vi "LogState.vi"(8 "error in (no error)":errorcluster, 10 "State In":string, 11 "String in":refnum<vi>) -> (0 "error out":errorcluster, 2 "State Out":string)   [LabVIEW 2017]
panel:
  out "Log line":string
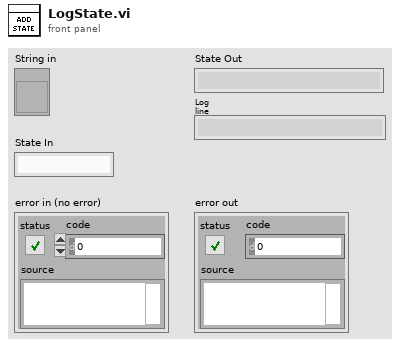
[diagram p1: front panel]
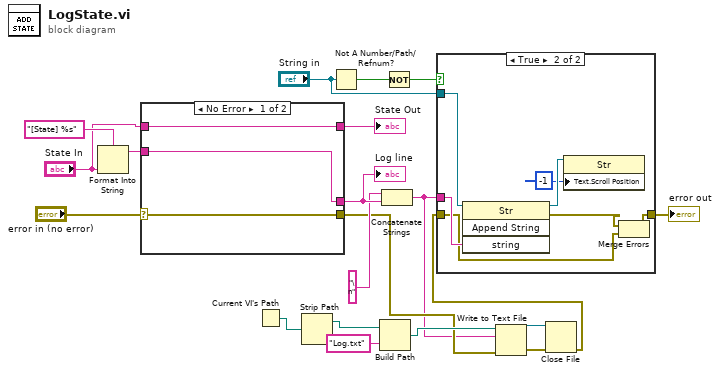
[diagram p0: block diagram]
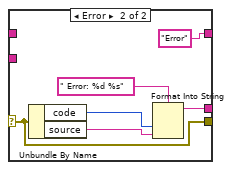
[diagram p3: hidden frame]
diagram:
  n1 = Format Into String(format string="[State] %s", "State In") -> (resulting string=w18:string)  [unwired: 2 in, 1 out]
  n2 = case shown="No Error" "error in (no error)" {
    selector: "error in (no error)" -> [w21 w24]
    tunnel: [w23 w26] -> w15
    tunnel: w18 -> [w23 _]
    tunnel: "State In" -> [w22 _]
    tunnel: [w22 "Error" ("State In")] -> w16
    tunnel: [w21 w24] -> w2
    frame No Error {
    }
    frame Error {
      n3 = Unbundle By Name(w24) -> ("code"=w28:i32, "source"=w27:string)
      n4 = Format Into String(format string=" Error: %d %s", w28, w27) -> (resulting string=w26:string)  [unwired: 2 in, 1 out]
    }
  }
  "State Out" <- w16
  "Log line" <- w15
  n5 = Current VI's Path() -> (path=w9:path)
  n6 = Strip Path(path=w9) -> (stripped path=w8:path)  [unwired: 1 out]
  n7 = Not A Number/Path/Refnum?(number/path/refnum="String in") -> (NaN/Path/Refnum?=w12:bool)
  n8 = Build Path(base path=w8, name or relative path="Log.txt") -> (appended path=w7:path)
  n9 = Concatenate Strings("\n" ("string"), w15) -> (w1:string)
  n10 = Not(x=w12) -> (.not. x?=w11:bool)
  n11 = Write to Text File(file (use dialog)=w7, text=w1, error in=w2) -> (refnum out=w6:refnum<file>, error out=w5:errorcluster)  [unwired: 1 in, 1 out]
  n12 = Close File(refnum=w6, error in=w5) -> (error out=w3:errorcluster)  [unwired: 1 out]
  n13 = case shown="True" w11 {
    tunnel: w1 -> [_ w37]
    tunnel: w3 -> [w30 w33]
    tunnel: [w30 w34] -> w13
    tunnel: "String in" -> [_ w36]
    frame False {
    }
    frame True {
      n14 = invoke class="Str" method="Append String"(reference=w36, "string"=w37) -> (reference out=w32:refnum<vi>, error out=w35:errorcluster)  [unwired: 2 in, 2 out]
      n15 = property class="Str"(reference=w32, "Text.Scroll Position"=-1) -> ()  [unwired: 1 in, 2 out]
      n16 = Merge Errors(w35, w33) -> (w34:errorcluster)
    }
  }
  "error out" <- w13
